vi "TCP客户端.vi"() -> ()   [LabVIEW 2018]
panel:
  in  "IP地址":string
  in  "接收区":string
  in  "发送区":string
  in  "连接":bool
  in  "停止":bool
  in  "读取":bool
  in  "发送":bool
  # "使用LABVIEW创建TCP客户端"
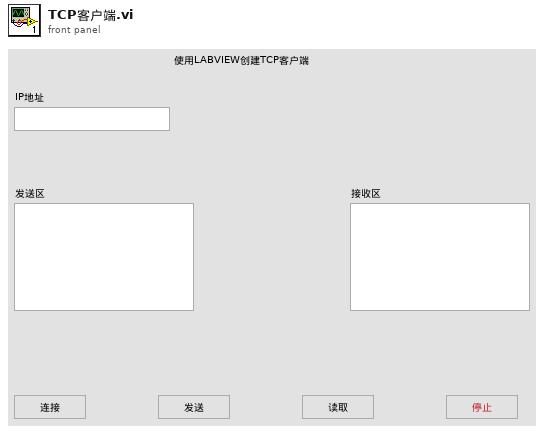
[diagram p1: front panel]
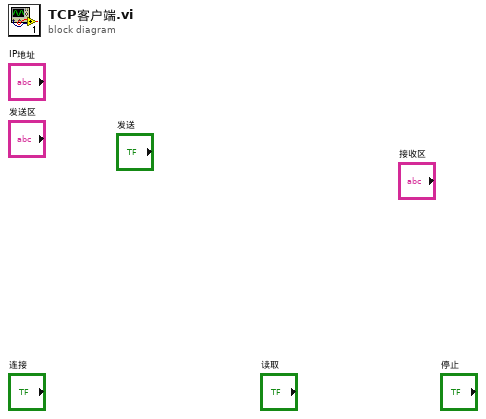
[diagram p0: block diagram]
diagram:
